vi "configure tls context.vi"(8 "error in":errorcluster, 10 "config":u64, 11 "context":u64) -> (0 "error out":errorcluster)   [LabVIEW 2016, in "lv tls dll.lvlib"]
uses:
  lv tls dll.lvlib
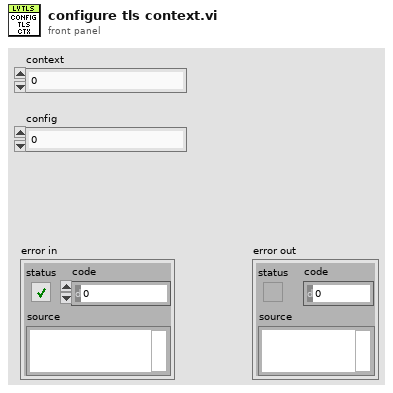
[diagram p1: front panel]
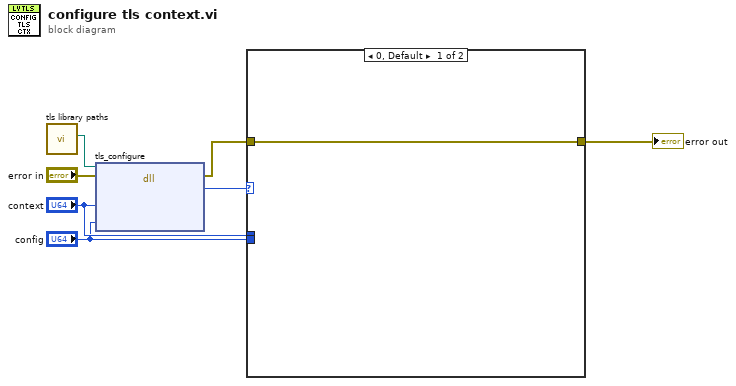
[diagram p0: block diagram]
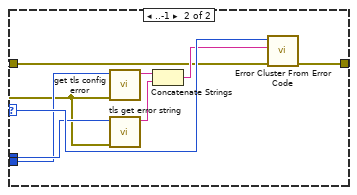
[diagram p2: hidden frame]
diagram:
  n1 = call "tls library paths.vi"() -> ("libtls"=w6:path)  [unwired: 8 in, 3 out]
  n2 = dll-call lib="C:/Users/IEUser/Desktop/tlssimple/libtls-15.dll" fn="tls_configure"(path in=w6, error in="error in", "context"="context", "config"="config") -> (error out=w1:errorcluster, "err"=w7:i32)  [unwired: 3 in, 1 out]
  n3 = case shown="0, Default" w7 {
    selector: w7 -> [_ w16]
    tunnel: [w8 w15] -> w4
    tunnel: "context" -> [_ w11]
    tunnel: "config" -> [_ w10]
    tunnel: w1 -> [w8 w9]
    frame 0, Default {
    }
    frame ..-1 {
      n4 = call "get tls config error.vi"("error in"=w9, "config"=w10) -> ("errString"=w13:string)  [unwired: 8 in, 1 out]
      n5 = call "tls get error string.vi"("error in"=w9, "tls context"=w11) -> ("error string"=w14:string)  [unwired: 8 in, 1 out]
      n6 = Concatenate Strings(w13, w14) -> (w12:string)
      n7 = call <vilib>:"Error Cluster From Error Code.vi"("error in (no error)"=w9, "error message (\"\")"=w12, "error code (0)"=w16) -> ("error out"=w15:errorcluster)  [unwired: 6 in]
    }
  }
  "error out" <- w4
